vi "Molar_mass_AIR_2022.vi"(8 "CO2 content (ppm)":dbl=542.0, 10 "xw molar fraction of water vapor":dbl=0.013091059810824573 format="%.6g", 11 "Type of air":i32(listbox)=4) -> (0 "xCH4":dbl=1.999543856771026e-06 format="%_3g", 1 "xKr":dbl=1.139739998359485e-06 format="%_4g", 2 "xHe":dbl=5.238804904740088e-06 format="%_5g", 3 "xNe":dbl=1.8175853658048626e-05 format="%_6g", 4 "xCO2":dbl=0.000542 format="%_6g", 5 "xN2":dbl=0.780661912560544 format="%_7g", 6 "xAr":dbl=0.009337869811120692 format="%.7g", 7 "xO2":dbl=0.20942822447048373 format="%_7g", 9 "Molar mass humid air [kg/mol]":dbl=0.028824480840518675 format="%#_7g")   [LabVIEW 2016]
panel:
  in  "Molar mass H2O":dbl=0.018015144 format="%#_13g"
  in  "Molar mass CH4":dbl=0.016042433 format="%#_13g"
  in  "Molar mass Kr":dbl=0.083798 format="%#_13g"
  in  "Molar mass He":dbl=0.004002602 format="%#_13g"
  in  "Molar mass Ne":dbl=0.0201797 format="%#_13g"
  in  "Molar Mass CO2":dbl=0.044010012 format="%#_13g"
  in  "Molar mass Ar":dbl=0.03995 format="%#_13g"
  in  "Molar mass O2":dbl=0.031998609 format="%#_13g"
  in  "Molar mass N2":dbl=0.028013452 format="%#_13g"
  out "Molar mass dry fraction [g/mol]":dbl=28.967863547202292 format="%_7g"
  out "differs from unity by (ppm)":dbl=-3.439215433553855 format="%.2g"
  out "total fraction check unity":dbl=0.9999965607845664
  out "Molar mass humid air [g/mol]":dbl=28.824480840518675 format="%_7g"
  # "molar masses in kg/mol from IUPAC atomic weights including natural variations updated 2022:\nfor N2 and O2 value for atmospheric air; for Ar updated value 2022; for CO2: C and O nat. var. in CO2; for He, Ne, Kr updated 2022; for CH4: C and H nat var in CH4; for H2O: H and O nat. var. in natural/continental water"
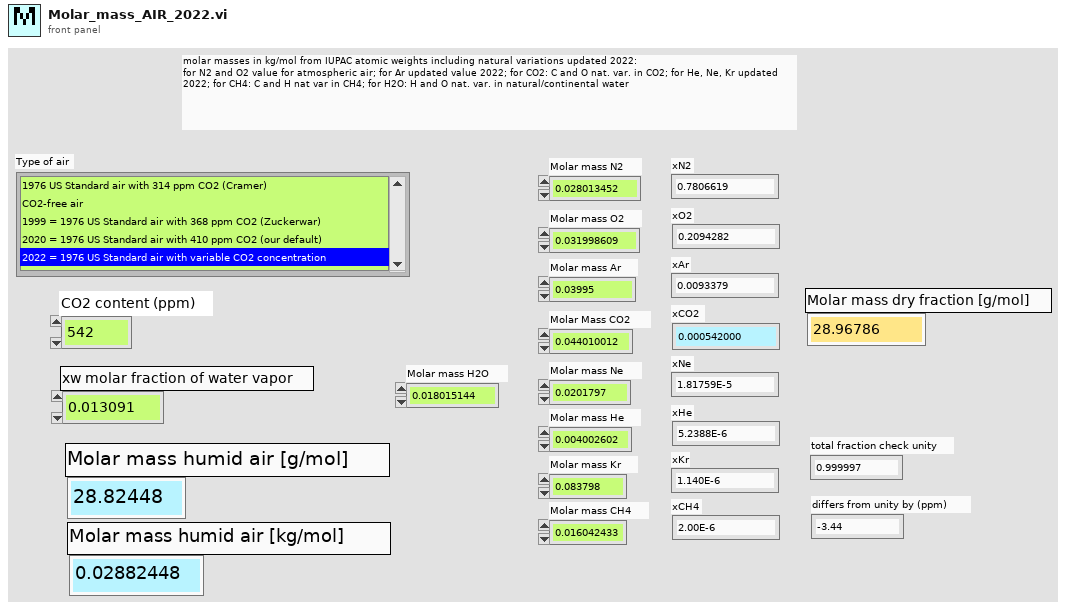
[diagram p1: front panel]
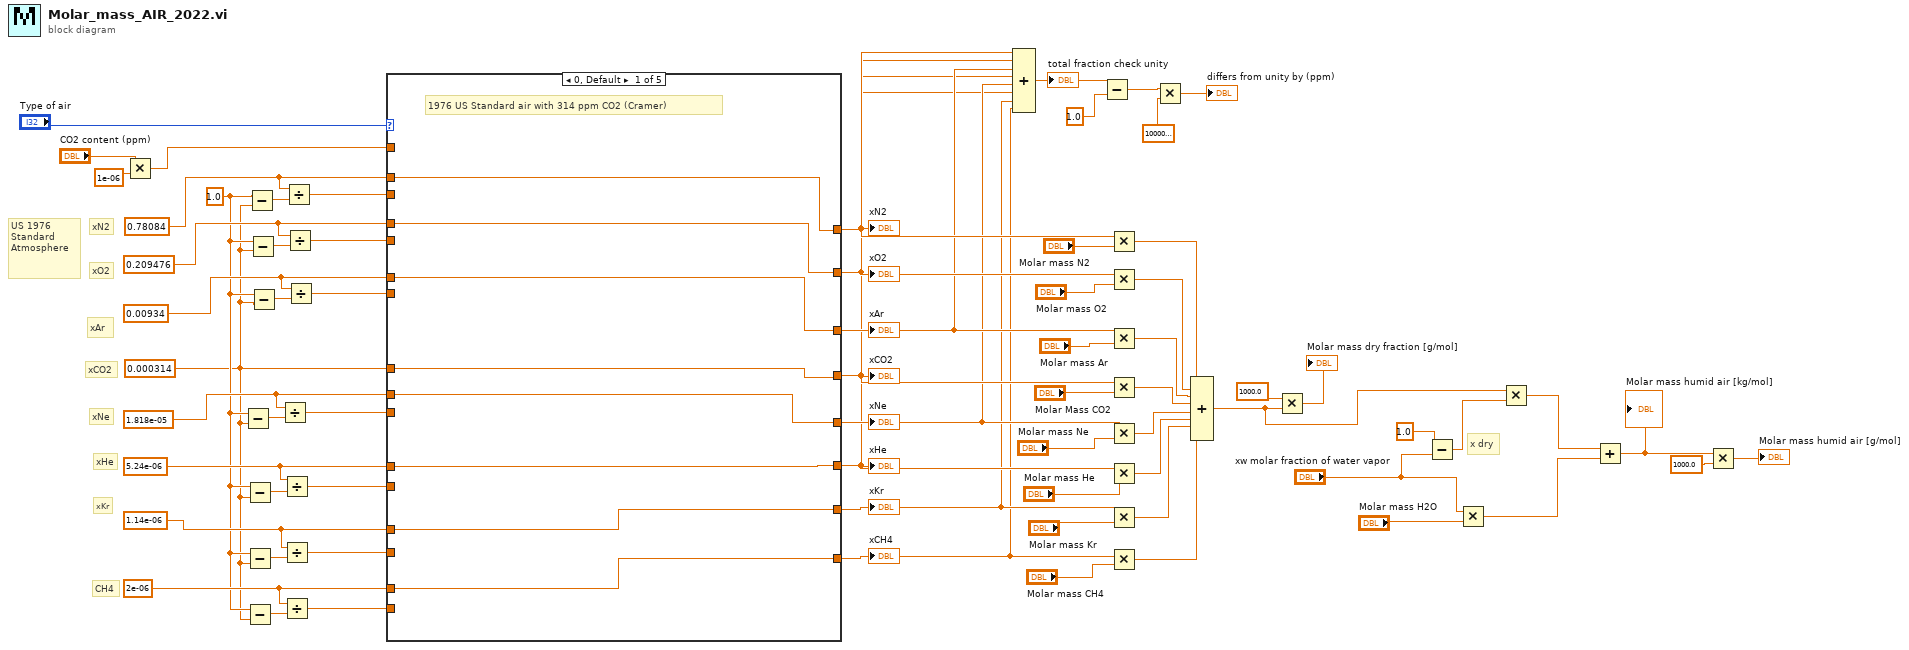
[diagram p0: block diagram]
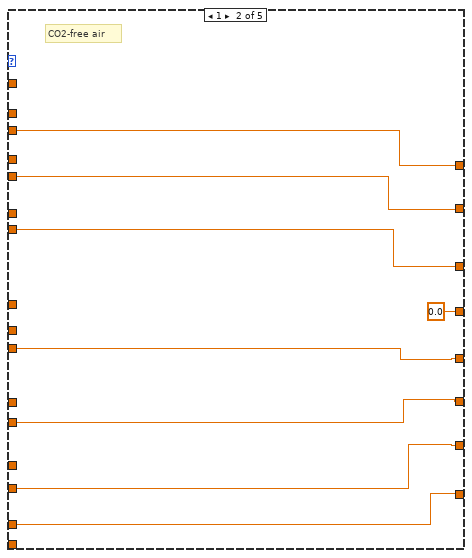
[diagram p2: hidden frame]
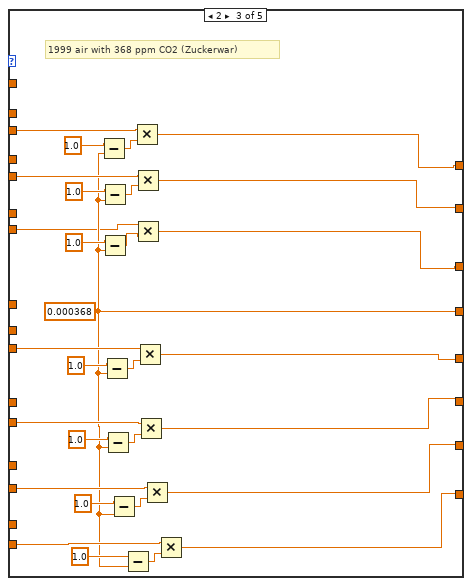
[diagram p3: hidden frame]
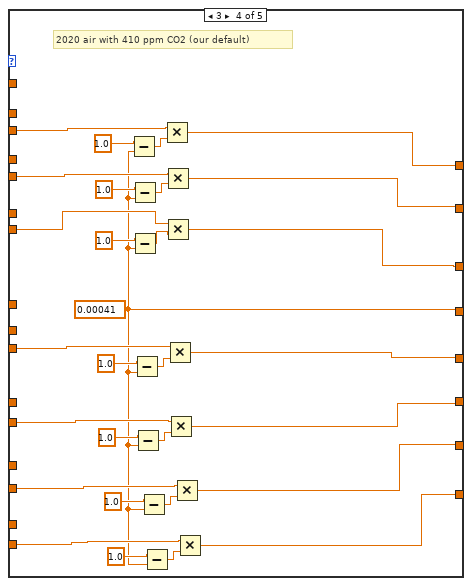
[diagram p4: hidden frame]
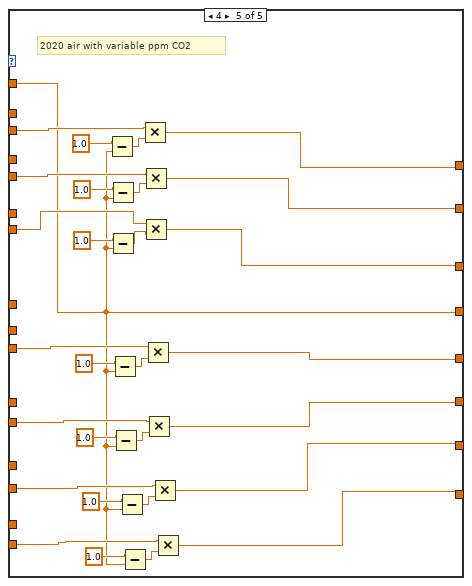
[diagram p5: hidden frame]
diagram:
  w23 = 0.000314
  w28 = 1.0 ("x")
  w29 = 2e-06
  w30 = 1.14e-06
  w31 = 5.24e-06
  w32 = 1.818e-05
  w40 = 0.00934
  w39 = 0.209476
  w44 = 0.78084
  # "x dry"
  # "CH4"
  # "xKr"
  # "xHe"
  # "xNe"
  # "xCO2"
  # "xAr"
  # "xO2"
  # "xN2"
  # "US 1976\nStandard\nAtmosphere"
  n1 = Multiply(x="CO2 content (ppm)", y=1e-06) -> (x*y=w63:dbl)
  n2 = Subtract(x=w28, y=w23) -> (x-y=w36:dbl)
  n3 = Subtract(x=w28, y=w23) -> (x-y=w35:dbl)
  n4 = Subtract(x=w28, y=w23) -> (x-y=w34:dbl)
  n5 = Subtract(x=w28, y=w23) -> (x-y=w33:dbl)
  n6 = Subtract(x=w28, y=w23) -> (x-y=w45:dbl)
  n7 = Subtract(x=w28, y=w23) -> (x-y=w42:dbl)
  n8 = Subtract(x=w28, y=w23) -> (x-y=w41:dbl)
  n9 = Divide(x=w32, y=w36) -> (x/y=w27:dbl)
  n10 = Divide(x=w31, y=w35) -> (x/y=w26:dbl)
  n11 = Divide(x=w30, y=w34) -> (x/y=w25:dbl)
  n12 = Divide(x=w29, y=w33) -> (x/y=w24:dbl)
  n13 = Divide(x=w44, y=w45) -> (x/y=w43:dbl)
  n14 = Divide(x=w39, y=w42) -> (x/y=w38:dbl)
  n15 = Divide(x=w40, y=w41) -> (x/y=w37:dbl)
  n16 = case shown="0, Default" "Type of air" {
    tunnel: [w76 w83 w99 w121 w145] -> w22
    tunnel: [w70 w82 w98 w120 w144] -> w21
    tunnel: [w75 w81 w97 w119 w143] -> w20
    tunnel: [w69 0.0 w86 w114 w150] -> w19
    tunnel: [w74 w80 w90 w118 w149] -> w18
    tunnel: [w73 w79 w89 w117 w148] -> w17
    tunnel: [w72 w78 w88 w116 w147] -> w16
    tunnel: [w71 w77 w87 w115 w146] -> w15
    tunnel: w63 -> [_ _ _ _ w150]
    tunnel: w44 -> [w76 _ _ _ _]
    tunnel: w39 -> [w70 _ _ _ _]
    tunnel: w40 -> [w75 _ _ _ _]
    tunnel: w32 -> [w74 _ _ _ _]
    tunnel: w31 -> [w73 _ _ _ _]
    tunnel: w30 -> [w72 _ _ _ _]
    tunnel: w29 -> [w71 w77 _ _ _]
    tunnel: w43 -> [_ w83 w110 w128 w157]
    tunnel: w38 -> [_ w82 w107 w127 w156]
    tunnel: w37 -> [_ w81 w85 w126 w155]
    tunnel: w27 -> [_ w80 w96 w125 w154]
    tunnel: w26 -> [_ w79 w93 w124 w153]
    tunnel: w25 -> [_ w78 w92 w123 w152]
    tunnel: w24 -> [_ _ w91 w122 w151]
    tunnel: w23 -> [w69 _ _ _ _]
    frame 0, Default {
      # "1976 US Standard air with 314 ppm CO2 (Cramer)"
    }
    frame 1 {
      # "CO2-free air"
    }
    frame 2 {
      w86 = 0.000368
      # "1999 air with 368 ppm CO2 (Zuckerwar)"
      n17 = Subtract(x=1.0, y=w86) -> (x-y=w109:dbl)
      n18 = Subtract(x=1.0, y=w86) -> (x-y=w108:dbl)
      n19 = Subtract(x=1.0, y=w86) -> (x-y=w106:dbl)
      n20 = Subtract(x=1.0, y=w86) -> (x-y=w104:dbl)
      n21 = Subtract(x=1.0, y=w86) -> (x-y=w102:dbl)
      n22 = Subtract(x=1.0, y=w86) -> (x-y=w100:dbl)
      n23 = Subtract(x=1.0, y=w86) -> (x-y=w94:dbl)
      n24 = Multiply(x=w110, y=w109) -> (x*y=w99:dbl)
      n25 = Multiply(x=w107, y=w108) -> (x*y=w98:dbl)
      n26 = Multiply(x=w85, y=w106) -> (x*y=w97:dbl)
      n27 = Multiply(x=w96, y=w104) -> (x*y=w90:dbl)
      n28 = Multiply(x=w93, y=w102) -> (x*y=w89:dbl)
      n29 = Multiply(x=w92, y=w100) -> (x*y=w88:dbl)
      n30 = Multiply(x=w91, y=w94) -> (x*y=w87:dbl)
    }
    frame 3 {
      w114 = 0.00041
      # "2020 air with 410 ppm CO2 (our default)"
      n31 = Subtract(x=1.0, y=w114) -> (x-y=w139:dbl)
      n32 = Subtract(x=1.0, y=w114) -> (x-y=w138:dbl)
      n33 = Subtract(x=1.0, y=w114) -> (x-y=w137:dbl)
      n34 = Subtract(x=1.0, y=w114) -> (x-y=w135:dbl)
      n35 = Subtract(x=1.0, y=w114) -> (x-y=w133:dbl)
      n36 = Subtract(x=1.0, y=w114) -> (x-y=w131:dbl)
      n37 = Subtract(x=1.0, y=w114) -> (x-y=w129:dbl)
      n38 = Multiply(x=w128, y=w139) -> (x*y=w121:dbl)
      n39 = Multiply(x=w127, y=w138) -> (x*y=w120:dbl)
      n40 = Multiply(x=w126, y=w137) -> (x*y=w119:dbl)
      n41 = Multiply(x=w125, y=w135) -> (x*y=w118:dbl)
      n42 = Multiply(x=w124, y=w133) -> (x*y=w117:dbl)
      n43 = Multiply(x=w123, y=w131) -> (x*y=w116:dbl)
      n44 = Multiply(x=w122, y=w129) -> (x*y=w115:dbl)
    }
    frame 4 {
      # "2020 air with variable ppm CO2"
      n45 = Subtract(x=1.0, y=w150) -> (x-y=w168:dbl)
      n46 = Subtract(x=1.0, y=w150) -> (x-y=w167:dbl)
      n47 = Subtract(x=1.0, y=w150) -> (x-y=w166:dbl)
      n48 = Subtract(x=1.0, y=w150) -> (x-y=w164:dbl)
      n49 = Subtract(x=1.0, y=w150) -> (x-y=w162:dbl)
      n50 = Subtract(x=1.0, y=w150) -> (x-y=w160:dbl)
      n51 = Subtract(x=1.0, y=w150) -> (x-y=w158:dbl)
      n52 = Multiply(x=w157, y=w168) -> (x*y=w145:dbl)
      n53 = Multiply(x=w156, y=w167) -> (x*y=w144:dbl)
      n54 = Multiply(x=w155, y=w166) -> (x*y=w143:dbl)
      n55 = Multiply(x=w154, y=w164) -> (x*y=w149:dbl)
      n56 = Multiply(x=w153, y=w162) -> (x*y=w148:dbl)
      n57 = Multiply(x=w152, y=w160) -> (x*y=w147:dbl)
      n58 = Multiply(x=w151, y=w158) -> (x*y=w146:dbl)
    }
  }
  "xN2" <- w22
  "xO2" <- w21
  "xAr" <- w20
  "xCO2" <- w19
  "xNe" <- w18
  "xHe" <- w17
  "xKr" <- w16
  "xCH4" <- w15
  n59 = Compound Arithmetic op=ADD(w22, w21, w20, w19, w18, w17, w16, w15) -> (w50:dbl)
  "total fraction check unity" <- w50
  n60 = Subtract(x=w50, y=1.0) -> (x-y=w47:dbl)
  n61 = Multiply(x=w22, y="Molar mass N2") -> (x*y=w14:dbl)
  n62 = Multiply(x=w21, y="Molar mass O2") -> (x*y=w12:dbl)
  n63 = Multiply(x=w20, y="Molar mass Ar") -> (x*y=w11:dbl)
  n64 = Multiply(x=w19, y="Molar Mass CO2") -> (x*y=w10:dbl)
  n65 = Multiply(x=w18, y="Molar mass Ne") -> (x*y=w9:dbl)
  n66 = Multiply(x=w17, y="Molar mass He") -> (x*y=w8:dbl)
  n67 = Multiply(x=w16, y="Molar mass Kr") -> (x*y=w7:dbl)
  n68 = Multiply(x=w15, y="Molar mass CH4") -> (x*y=w13:dbl)
  n69 = Multiply(x=w47, y=1000000.0) -> (x*y=→"differs from unity by (ppm)":dbl)
  n70 = Compound Arithmetic op=ADD(w14, w12, w11, w10, w9, w8, w7, w13) -> (w3:dbl)
  n71 = Multiply(x=1000.0, y=w3) -> (x*y=→"Molar mass dry fraction [g/mol]":dbl)
  n72 = Subtract(x=1.0, y="xw molar fraction of water vapor") -> (x-y=w66:dbl)
  n73 = Multiply(x="xw molar fraction of water vapor", y="Molar mass H2O") -> (x*y=w4:dbl)
  n74 = Multiply(x=w3, y=w66) -> (x*y=w5:dbl)
  n75 = Add(x=w5, y=w4) -> (x+y=w2:dbl)
  "Molar mass humid air [kg/mol]" <- w2
  n76 = Multiply(x=w2, y=1000.0) -> (x*y=→"Molar mass humid air [g/mol]":dbl)
